vi "Localization.vi"(11 "Motors":T1={"Drive Motors (NEO)"={"Left Front"={"DeviceStatus"={"status"=FALSE, "code"=0, "source"=""}, "Type"=enum."PWM", "PWM"={"PWM Channel"=enum."Invalid", "DeadBand"={"Name"="", "maxPositivePwm"=0, "minPositivePwm"=0, "centerPwm"=0, "maxNegativePwm"=0, "minNegativePwm"=0, "angularRange"=0}}, "CAN"={"Device Number"=0, "SetOutput VI Ref"=variant, "GetOutput VI Ref"=variant, "Enable VI Ref"=variant, "Disable VI Ref"=variant, "Data"=variant}, "Invert"=FALSE, "DIO PWM"={"PWM \"Enable\" Channel"=enum."Invalid", "DIOChannel"=enum."Invalid", "PWM Rate"=0.0}}, "Left Back"={"DeviceStatus"={"status"=FALSE, "code"=0, "source"=""}, "Type"=enum."PWM", "PWM"={"PWM Channel"=enum."Invalid", "DeadBand"={"Name"="", "maxPositivePwm"=0, "minPositivePwm"=0, "centerPwm"=0, "maxNegativePwm"=0, "minNegativePwm"=0, "angularRange"=0}}, "CAN"={"Device Number"=0, "SetOutput VI Ref"=variant, "GetOutput VI Ref"=variant, "Enable VI Ref"=variant, "Disable VI Ref"=variant, "Data"=variant}, "Invert"=FALSE, "DIO PWM"={"PWM \"Enable\" Channel"=enum."Invalid", "DIOChannel"=enum."Invalid", "PWM Rate"=0.0}}, "Right Front"={"DeviceStatus"={"status"=FALSE, "code"=0, "source"=""}, "Type"=enum."PWM", "PWM"={"PWM Channel"=enum."Invalid", "DeadBand"={"Name"="", "maxPositivePwm"=0, "minPositivePwm"=0, "centerPwm"=0, "maxNegativePwm"=0, "minNegativePwm"=0, "angularRange"=0}}, "CAN"={"Device Number"=0, "SetOutput VI Ref"=variant, "GetOutput VI Ref"=variant, "Enable VI Ref"=variant, "Disable VI Ref"=variant, "Data"=variant}, "Invert"=FALSE, "DIO PWM"={"PWM \"Enable\" Channel"=enum."Invalid", "DIOChannel"=enum."Invalid", "PWM Rate"=0.0}}, "Right Back"={"DeviceStatus"={"status"=FALSE, "code"=0, "source"=""}, "Type"=enum."PWM", "PWM"={"PWM Channel"=enum."Invalid", "DeadBand"={"Name"="", "maxPositivePwm"=0, "minPositivePwm"=0, "centerPwm"=0, "maxNegativePwm"=0, "minNegativePwm"=0, "angularRange"=0}}, "CAN"={"Device Number"=0, "SetOutput VI Ref"=variant, "GetOutput VI Ref"=variant, "Enable VI Ref"=variant, "Disable VI Ref"=variant, "Data"=variant}, "Invert"=FALSE, "DIO PWM"={"PWM \"Enable\" Channel"=enum."Invalid", "DIOChannel"=enum."Invalid", "PWM Rate"=0.0}}}, "Steer Motors (NEO)"={"Left Front"={"DeviceStatus"={"status"=FALSE, "code"=0, "source"=""}, "Type"=enum."PWM", "PWM"={"PWM Channel"=enum."Invalid", "DeadBand"={"Name"="", "maxPositivePwm"=0, "minPositivePwm"=0, "centerPwm"=0, "maxNegativePwm"=0, "minNegativePwm"=0, "angularRange"=0}}, "CAN"={"Device Number"=0, "SetOutput VI Ref"=variant, "GetOutput VI Ref"=variant, "Enable VI Ref"=variant, "Disable VI Ref"=variant, "Data"=variant}, "Invert"=FALSE, "DIO PWM"={"PWM \"Enable\" Channel"=enum."Invalid", "DIOChannel"=enum."Invalid", "PWM Rate"=0.0}}, "Left Back"={"DeviceStatus"={"status"=FALSE, "code"=0, "source"=""}, "Type"=enum."PWM", "PWM"={"PWM Channel"=enum."Invalid", "DeadBand"={"Name"="", "maxPositivePwm"=0, "minPositivePwm"=0, "centerPwm"=0, "maxNegativePwm"=0, "minNegativePwm"=0, "angularRange"=0}}, "CAN"={"Device Number"=0, "SetOutput VI Ref"=variant, "GetOutput VI Ref"=variant, "Enable VI Ref"=variant, "Disable VI Ref"=variant, "Data"=variant}, "Invert"=FALSE, "DIO PWM"={"PWM \"Enable\" Channel"=enum."Invalid", "DIOChannel"=enum."Invalid", "PWM Rate"=0.0}}, "Right Front"={"DeviceStatus"={"status"=FALSE, "code"=0, "source"=""}, "Type"=enum."PWM", "PWM"={"PWM Channel"=enum."Invalid", "DeadBand"={"Name"="", "maxPositivePwm"=0, "minPositivePwm"=0, "centerPwm"=0, "maxNegativePwm"=0, "minNegativePwm"=0, "angularRange"=0}}, "CAN"={"Device Number"=0, "SetOutput VI Ref"=variant, "GetOutput VI Ref"=variant, "Enable VI Ref"=variant, "Disable VI Ref"=variant, "Data"=variant}, "Invert"=FALSE, "DIO PWM"={"PWM \"Enable\" Channel"=enum."Invalid", "DIOChannel"=enum."Invalid", "PWM Rate"=0.0}}, "Right Back"={"DeviceStatus"={"status"=FALSE, "code"=0, "source"=""}, "Type"=enum."PWM", "PWM"={"PWM Channel"=enum."Invalid", "DeadBand"={"Name"="", "maxPositivePwm"=0, "minPositivePwm"=0, "centerPwm"=0, "maxNegativePwm"=0, "minNegativePwm"=0, "angularRange"=0}}, "CAN"={"Device Number"=0, "SetOutput VI Ref"=variant, "GetOutput VI Ref"=variant, "Enable VI Ref"=variant, "Disable VI Ref"=variant, "Data"=variant}, "Invert"=FALSE, "DIO PWM"={"PWM \"Enable\" Channel"=enum."Invalid", "DIOChannel"=enum."Invalid", "PWM Rate"=0.0}}}, "PigeonIMUDevRef"={"DeviceStatus"={"status"=FALSE, "code"=0, "source"=""}, "Device Number"=0, "Type"=352321536, "Device ID"=0, "Handle"=0, "UsageFrame"=0, "Library Path"=path ""}, "Radii (ft)"={"Left Front Position"=[], "Left Back Position"=[], "Right Front Position"=[], "Right Back Position"=[]}} {"Radii (ft)"."Right Back Position" format="%.2f"; "Radii (ft)"."Right Front Position" format="%.2f"; "Radii (ft)"."Left Back Position" format="%.2f"; "Radii (ft)"."Left Front Position" format="%.2f"; "PigeonIMUDevRef"."Type" items=["CAN"=352321536, "TalonSRX"=33554432]}) -> (2 "Y":dbl, 3 "X":dbl)   [LabVIEW 2025]
uses:
  swerve-template/Type Definitions/Hardware/Swerve Drives/(NEO-NEO-ThroughBore-Pigeon2) Swerve.ctl
  swerve-template/Type Definitions/Hardware/4 Motor Sets/(NEO & NEO 550) 4 Motor Set.ctl
  <vilib>/Rock Robotics/WPI/MotorControl/WPI_MotorControlDeviceRef.ctl
  <vilib>/Rock Robotics/WPI/MotorControl/WPI_MotorControlType.ctl
  <vilib>/Rock Robotics/SystemInterfaces/DIO/FPGA_DIOPWMChannel.ctl
  <vilib>/Rock Robotics/WPI/PWM/WPI_PWMDeadband.ctl
  <vilib>/Rock Robotics/SystemInterfaces/DIO/FPGA_DIOChannel.ctl
  <vilib>/Rock Robotics/WPI/ThirdParty/Phoenix-LabVIEW/Pigeon IMU/CTRE_PigeonIMU_DeviceRef.ctl
  <vilib>/Rock Robotics/WPI/ThirdParty/Phoenix-LabVIEW/Pigeon IMU/CTRE_PigeonIMU_ConnectionType.ctl
  swerve-template/Type Definitions/Data/Pod Positions.ctl
  <vilib>/Rock Robotics/WPI/DriverStation/WPI_DriverStationAllianceInfo.ctl
  <vilib>/Rock Robotics/Network Tables/NT Read Numeric Array.vi
  <vilib>/Rock Robotics/Network Tables/NT Read Number.vi
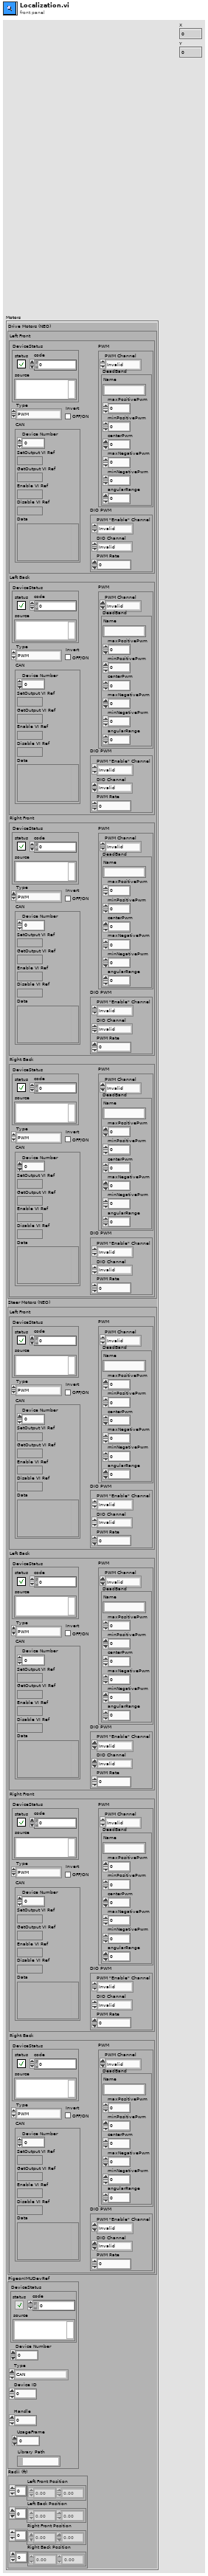
[diagram p1: front panel]
types:
  T1 = typedef "(NEO-NEO-ThroughBore-Pigeon2) Swerve.ctl" = cluster{"Drive Motors (NEO)":T2, "Steer Motors (NEO)":T2, "PigeonIMUDevRef":T8, "Radii (ft)":T10}
  T2 = typedef "(NEO & NEO 550) 4 Motor Set.ctl" = cluster{"Left Front":T3, "Left Back":T3, "Right Front":T3, "Right Back":T3}
  T3 = typedef "WPI_MotorControlDeviceRef.ctl" = cluster{"DeviceStatus":errorcluster, "Type":T4, "PWM":cluster{"PWM Channel":T5, "DeadBand":T6}, "CAN":cluster{"Device Number":u8, "SetOutput VI Ref":variant, "GetOutput VI Ref":variant, "Enable VI Ref":variant, "Disable VI Ref":variant, "Data":variant}, "Invert":bool, "DIO PWM":cluster{"PWM \"Enable\" Channel":T5, "DIOChannel":T7, "PWM Rate":dbl}}
  T4 = typedef "WPI_MotorControlType.ctl" = enum16{"PWM", "CAN", "DIO PWM"}
  T5 = typedef "FPGA_DIOPWMChannel.ctl" = enum8{"PWM 0", "PWM 1", "PWM 2", "PWM 3", "PWM 4", "PWM 5", "PWM 6", "PWM 7", "PWM 8", "PWM 9", "PWM MXP 0", "PWM MXP 1", "PWM MXP 2", "PWM MXP 3", "PWM MXP 4", "PWM MXP 5", "PWM MXP 6", "PWM MXP 7", "PWM MXP 8", "PWM MXP 9", "Invalid"}
  T6 = typedef "WPI_PWMDeadband.ctl" = cluster{"Name":string, "maxPositivePwm":i32, "minPositivePwm":i32, "centerPwm":i32, "maxNegativePwm":i32, "minNegativePwm":i32, "angularRange":u16}
  T7 = typedef "FPGA_DIOChannel.ctl" = enum8{"DIO 0", "DIO 1", "DIO 2", "DIO 3", "DIO 4", "DIO 5", "DIO 6", "DIO 7", "DIO 8", "DIO 9", "DIO MXP 0", "DIO MXP 1", "DIO MXP 2", "DIO MXP 3", "DIO MXP 4", "DIO MXP 5", "DIO MXP 6", "DIO MXP 7", "DIO MXP 8", "DIO MXP 9", "DIO MXP 10", "DIO MXP 11", "DIO MXP 12", "DIO MXP 13", "DIO MXP 14", "DIO MXP 15", "SPI Port CS1", "SPI Port CS2", "SPI Port CS3", "SPI Port MISO", "SPI Port MOSI", "Invalid"}
  T8 = typedef "CTRE_PigeonIMU_DeviceRef.ctl" = cluster{"DeviceStatus":errorcluster, "Device Number":u8, "Type":T9, "Device ID":u32, "Handle":u64, "UsageFrame":u32, "Library Path":path}
  T9 = typedef "CTRE_PigeonIMU_ConnectionType.ctl" = u32
  T10 = typedef "Pod Positions.ctl" = cluster{"Left Front Position":dbl[], "Left Back Position":dbl[], "Right Front Position":dbl[], "Right Back Position":dbl[]}
  T11 = typedef "WPI_DriverStationAllianceInfo.ctl" = enum16{"Red", "Blue", "Invalid"}
  T12 = cluster{"Left Front":dbl, "Left Back":dbl, "Right Front":dbl, "Right Back":dbl}
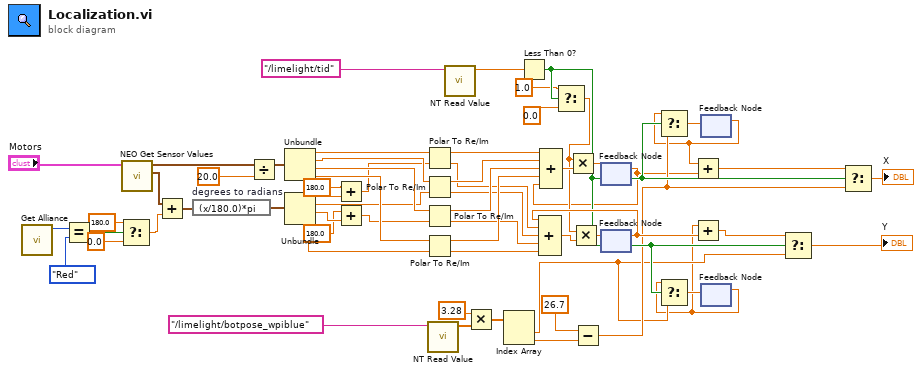
[diagram p0: block diagram]
diagram:
  n1 = call "Get Alliance.vi"() -> ("Alliance"=w7:T11)  [unwired: 11 in]
  n2 = Equal?(x=w7, y=WPI_DriverStationAllianceInfo."Red") -> (x = y?=w6:bool)
  n3 = Select(t=180.0, s=w6, f=0.0) -> (s? t:f=w2:dbl)
  n4 = call "NEO Get Sensor Values.vi"("Swerve Motors"="Motors") -> ("Steer Angles (degrees)"=w38:T12, "Drive Velocities (ft/s)"=w23:T12)  [unwired: 9 in]
  n5 = Add(x=w38, y=w2) -> (x+y=w37:T12)
  n6 = expression code="(x/180.0)*pi" "degrees to radians"(w37) -> (w36:T12)
  n7 = Divide(x=w23, y=20.0) -> (x/y=w21:T12)
  n8 = Unbundle(w21) -> ("Left Front"=w60:dbl, "Left Back"=w59:dbl, "Right Front"=w58:dbl, "Right Back"=w57:dbl)
  n9 = Unbundle(w36) -> ("Left Front"=w16:dbl, "Left Back"=w56:dbl, "Right Front"=w13:dbl, "Right Back"=w55:dbl)
  n10 = Add(x=180.0, y=w16) -> (x+y=w14:dbl)
  n11 = Add(x=180.0, y=w13) -> (x+y=w12:dbl)
  n12 = Polar To Re/Im(2:w14, 3:w60) -> (0:w47:dbl, 1:w54:dbl)
  n13 = Polar To Re/Im(2:w56, 3:w59) -> (0:w48:dbl, 1:w53:dbl)
  n14 = Polar To Re/Im(2:w12, 3:w58) -> (0:w49:dbl, 1:w52:dbl)
  n15 = Polar To Re/Im(2:w55, 3:w57) -> (0:w50:dbl, 1:w51:dbl)
  n16 = call-poly <vilib>:"NT Read Value.vi"("name"="/limelight/botpose_wpiblue") -> ("value"=w46:dbl[])  [unwired: 8 in, 2 out]
  n17 = call-poly <vilib>:"NT Read Value.vi"("name"="/limelight/tid") -> ("value"=w39:dbl)  [unwired: 8 in, 2 out]
  n18 = Multiply(x=3.28 ("Numeric"), y=w46) -> (x*y=w44:dbl[])
  n19 = Index Array(array=w44) -> (element #1=w17:dbl, element #2=w42:dbl)  [unwired: 2 in]
  n20 = Less Than 0?(x=w39) -> (x < 0?=w31:bool)
  n21 = Select(t=1.0, s=w31, f=0.0) -> (s? t:f=w24:dbl)
  n22 = Subtract(x=26.7, y=w42) -> (x-y=w18:dbl)
  n23 = feedback #1() -> (w9:dbl)  [unwired: 1 in]
  n24 = Compound Arithmetic op=ADD(w54, w53, w52, w51, w9) -> (w27:dbl)
  n25 = Multiply(x=w24, y=w27) -> (x*y=w28:dbl)
  n26 = feedback-in #1(w28) -> ()
  n27 = feedback #2() -> (w34:dbl)  [unwired: 1 in]
  n28 = Compound Arithmetic op=ADD(w34, w47, w48, w49, w50) -> (w25:dbl)
  n29 = Multiply(x=w24, y=w25) -> (x*y=w26:dbl)
  n30 = feedback-in #2(w26) -> ()
  n31 = feedback #3() -> (w10:dbl)  [unwired: 1 in]
  n32 = Select(t=w10, s=w31, f=w18) -> (s? t:f=w32:dbl)
  n33 = Add(x=w10, y=w9) -> (x+y=w1:dbl)
  n34 = feedback-in #3(w32) -> ()
  n35 = feedback #4() -> (w8:dbl)  [unwired: 1 in]
  n36 = Select(t=w8, s=w31, f=w17) -> (s? t:f=w33:dbl)
  n37 = Add(x=w8, y=w34) -> (x+y=w35:dbl)
  n38 = feedback-in #4(w33) -> ()
  n39 = Select(t=w35, s=w31, f=w17) -> (s? t:f=→"Y":dbl)
  n40 = Select(t=w1, s=w31, f=w18) -> (s? t:f=→"X":dbl)
